vi "IPI_Cal_Step1.vi"(10 "Program":string(combo)="potteryTemplete", 11 "Image In":T2) -> (1 "Piex":string, 2 "result":string, 3 "Image Out":T2(plugin-control))   [LabVIEW 2015]
uses:
  <vilib>/vision/Image Controls.llb/IMAQ Image.ctl
  Global System.vi
  <vilib>/Utility/file.llb/Read Delimited Spreadsheet (string).vi
  <vilib>/vision/driver/NI_Vision_Acquisition_Software.lvlib
  <vilib>/Analysis/NI_AALPro.lvlib
panel:
  out "数字":i32[](array[numeric])
  out "all rows":string[][](array[string]) caption="所有行"
  out "Straight Edge (Find Straight Edge 1) 2":T1 {"Point2 (Real-World)"."Y" format="%.2f"; "Point2 (Real-World)"."X" format="%.2f"; "Point1 (Real-World)"."Y" format="%.2f"; "Point1 (Real-World)"."X" format="%.2f"; "Point2 (Pixels)"."Y" format="%.2f"; "Point2 (Pixels)"."X" format="%.2f"; "Point1 (Pixels)"."Y" format="%.2f"; "Point1 (Pixels)"."X" format="%.2f"}
  out "输出簇":cluster{"X":i32, "Y":i32}
  out "Dist piex":dbl
  out "y 焦点":dbl
  out "X 焦点":dbl
  out "b2":dbl
  out "k2":dbl
  out "元素":cluster{"X":dbl, "Y":dbl}
  out "数组":dbl[](array[numeric])
  out "大小":i32
  out "Contour Points (Contour Analysis 1)":cluster{"X":dbl, "Y":dbl}[](array[cluster])
  out "b1":dbl caption="截距"
  out "k1":dbl caption="斜率"
  in  "error in":errorcluster
  out "Straight Edge (Find Straight Edge 1)":T1 {"Point2 (Real-World)"."Y" format="%.2f"; "Point2 (Real-World)"."X" format="%.2f"; "Point1 (Real-World)"."Y" format="%.2f"; "Point1 (Real-World)"."X" format="%.2f"; "Point2 (Pixels)"."Y" format="%.2f"; "Point2 (Pixels)"."X" format="%.2f"; "Point1 (Pixels)"."Y" format="%.2f"; "Point1 (Pixels)"."X" format="%.2f"}
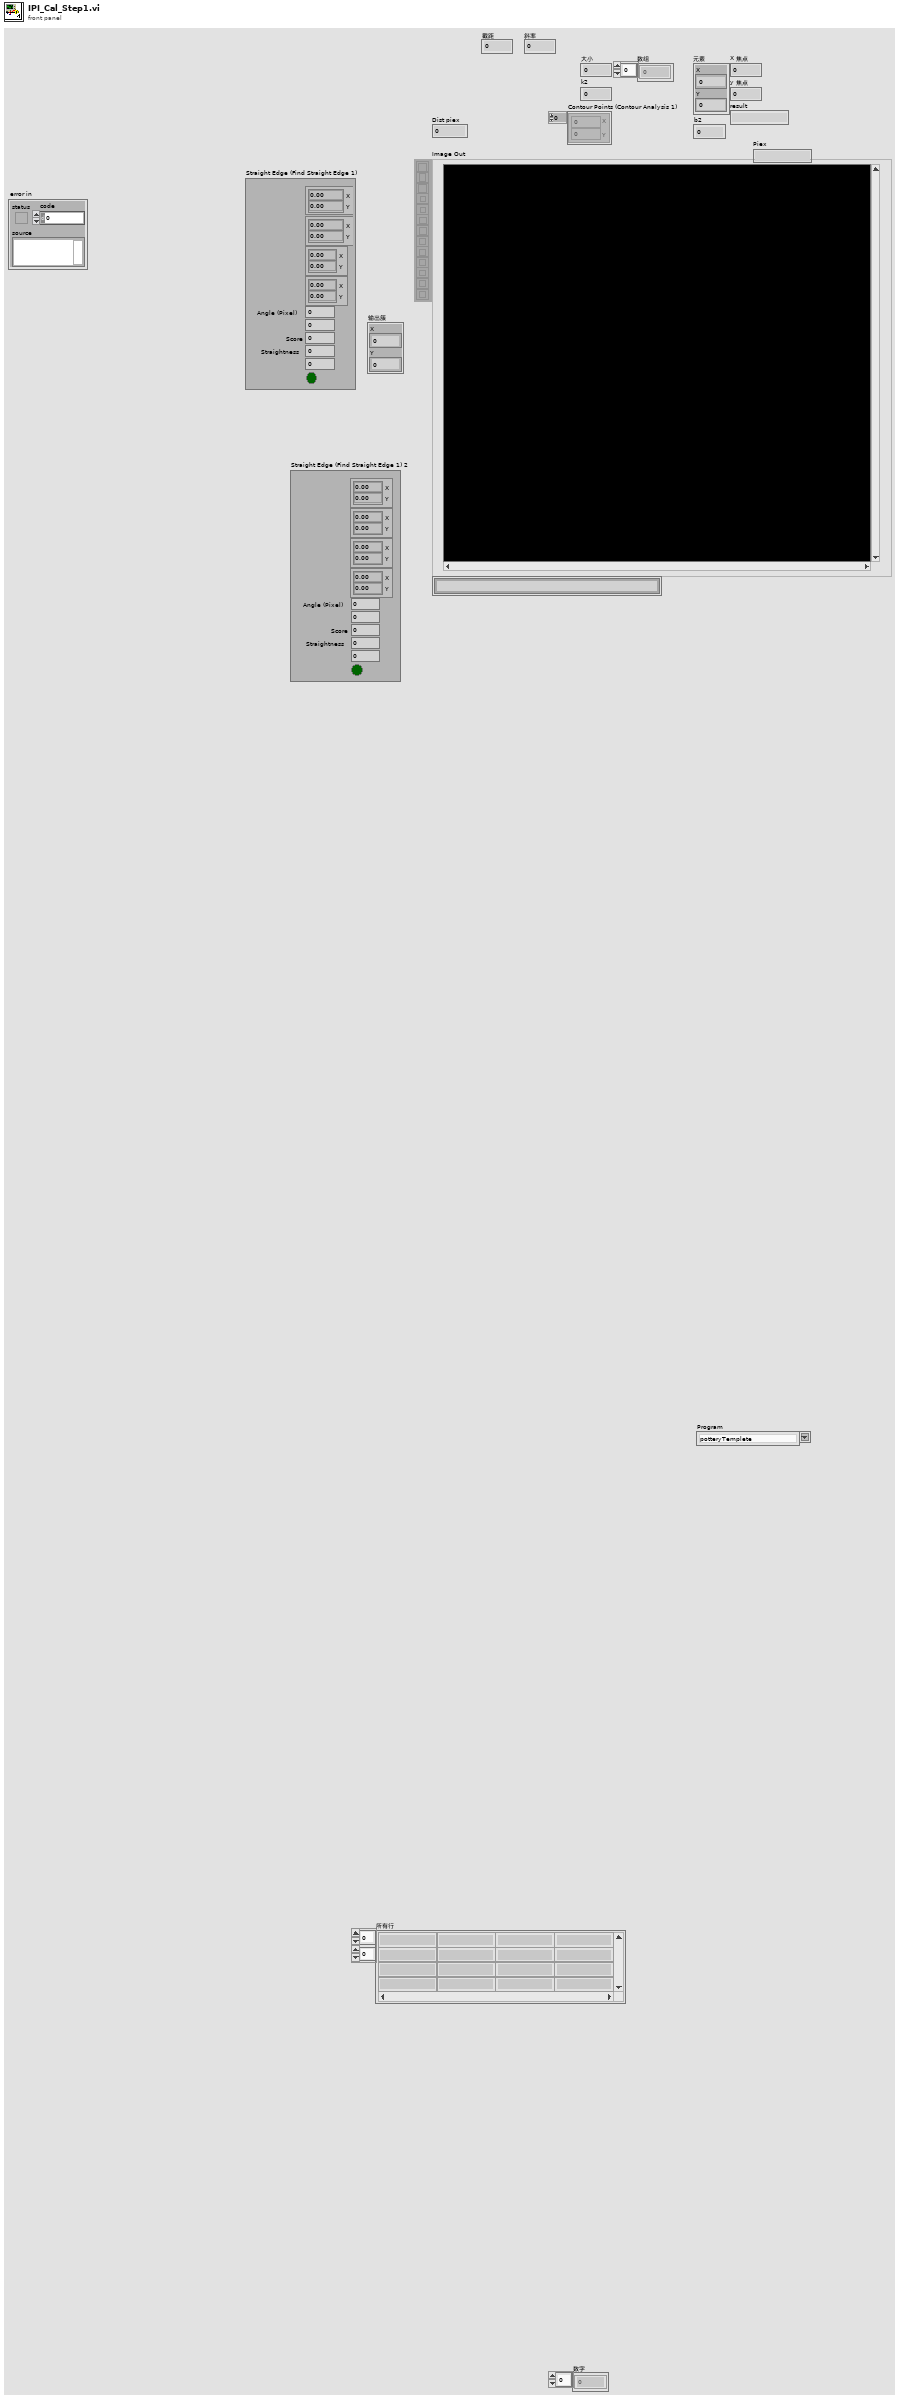
[diagram p1: front panel]
types:
  T1 = cluster{"Point1 (Pixels)":cluster{"X":sgl, "Y":sgl}, "Point2 (Pixels)":cluster{"X":sgl, "Y":sgl}, "Point1 (Real-World)":cluster{"X":sgl, "Y":sgl}, "Point2 (Real-World)":cluster{"X":sgl, "Y":sgl}, "Angle (Pixel)":dbl, "Angle (Real-World)":dbl, "Score":dbl, "Straightness":dbl, "Average SNR (db)":dbl, "Calibration Valid":bool}
  T2 = typedef "IMAQ Image.ctl" = refnum<image>
  T3 = cluster{"ID":enum32{"External", "Internal"}, "Type":u32, "Coordinates":i32[]}
  T4 = cluster{"Global Rectangle":i32[], "Contours":cluster{"ID":enum32{"External", "Internal"}, "Type":u32, "Coordinates":i32[]}[]}
  T5 = typedef "IMAQdx.ctl" = refnum<k21>
  T6 = cluster{"ID":enum32{"External", "Internal"}, "Type":u32, "Coordinates":i32[]}[]
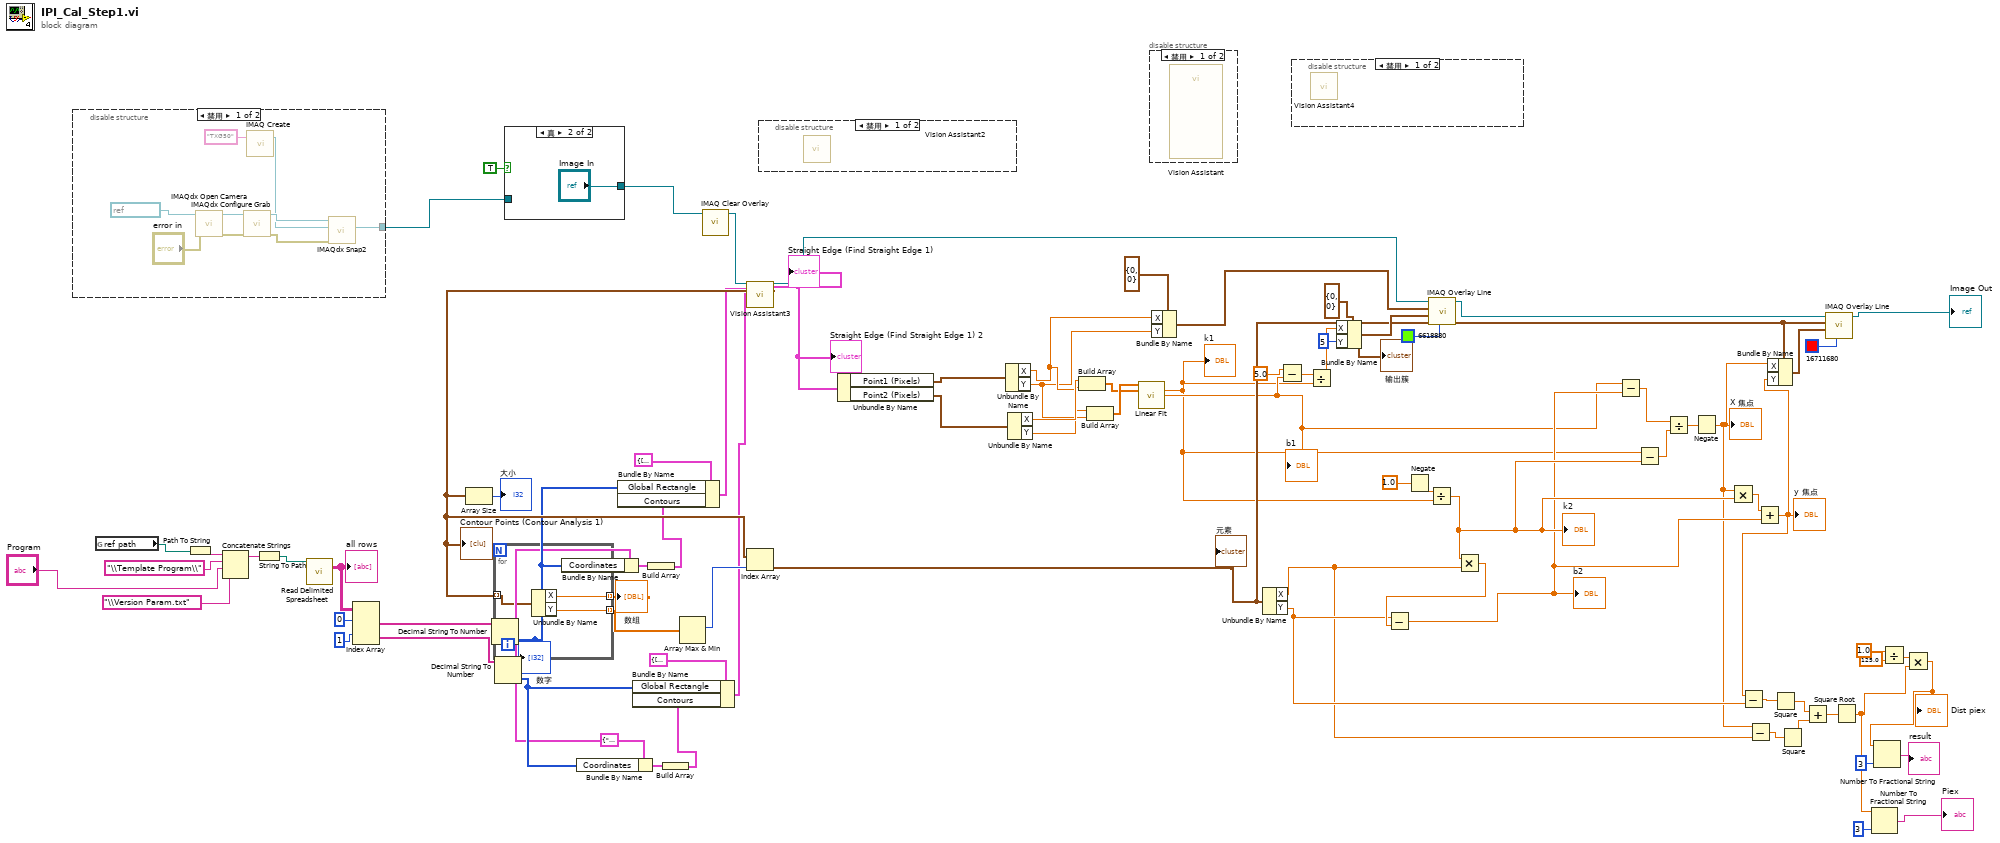
[diagram p0: block diagram]
diagram:
  w6 = T3 {"ID"=enum."External", "Type"=12, "Coordinates"=[983, 377, 1194, 1554, 1829]}
  n1 = disable-structure shown="禁用" {
    disable-tunnel: [w86 _] -> w4
    frame Disabled {
      n2 = call <vilib>:"IMAQdx Open Camera.vi"("error in"="error in", "Session In"=refnum<k21> "TXG50" ("Camera Name")) -> ("error out"=w94:errorcluster, "Session Out"=w93:T5)  [unwired: 1 in, 7 out]
      n3 = call <vilib>:"IMAQdx Configure Grab.vi"("error in"=w94, "Session In"=w93) -> ("error out"=w87:errorcluster, "Session Out"=w89:T5)  [unwired: 8 out]
      n4 = call "IMAQ Create"("Image Name"="TXG50") -> ("New Image"=w88:T2)  [unwired: 4 in, 1 out]
      n5 = call <vilib>:"IMAQdx Snap2.vi"("error in"=w87, "Image In"=w88, "Session In"=w89) -> ("Image Out"=w86:T2)  [unwired: 6 in, 2 out]
    }
    frame Enabled {
    }
  }
  n6 = global read "Global System.vi" "ref path"() -> (w23:path)
  n7 = Path To String(path=w23) -> (string=w25:string)
  n8 = Concatenate Strings(w25, "\\Template Program\\" ("字符串"), "Program", "\\Version Param.txt" ("字符串")) -> (w24:string)
  n9 = String To Path(string=w24) -> (path=w19:path)
  n10 = call-poly <vilib>:"Read Delimited Spreadsheet.vi"("file path (dialog if empty)"=w19) -> ("all rows"=w17:string[][])  [unwired: 9 in, 5 out]
  "all rows" <- w17
  n11 = Index Array(array=w17, index (row) #1=0 ("索引 (行)"), index (row) #2=1 ("禁用的索引 (列)")) -> (element #1=w16:string[], element #2=w11:string[])  [unwired: 2 in]
  n12 = Decimal String To Number(string=w16) -> (number=w13:i32[])  [unwired: 2 in, 1 out]
  "数字" <- w13
  n13 = Decimal String To Number(string=w11) -> (number=w8:i32[])  [unwired: 2 in, 1 out]
  n14 = case shown="真" TRUE {
    tunnel: [w95 "Image In"] -> w33
    tunnel: w4 -> [w95 _]
    frame False {
    }
    frame True {
    }
  }
  n15 = Bundle By Name(cluster=w6, "Coordinates"=w13) -> (w15:T3)
  n16 = Bundle By Name(cluster=w6, "Coordinates"=w8) -> (w10:T3)
  n17 = Build Array(w15) -> (w14:T6)
  n18 = Bundle By Name(cluster=T4 {"Global Rectangle"=[964, 373, 1213, 1558], "Contours"=[{"ID"=enum."External", "Type"=12, "Coordinates"=[983, 377, 1194, 1554, 1829]}]} ("ROI Descriptor (Find Straight Edge 1)"), "Global Rectangle"=w13, "Contours"=w14) -> (w5:T4)
  n19 = Build Array(w10) -> (w7:T6)
  n20 = Bundle By Name(cluster=T4 {"Global Rectangle"=[964, 373, 1213, 1558], "Contours"=[{"ID"=enum."External", "Type"=12, "Coordinates"=[983, 377, 1194, 1554, 1829]}]} ("ROI Descriptor (Find Straight Edge 1)"), "Global Rectangle"=w8, "Contours"=w7) -> (w1:T4)
  n21 = call "IMAQ Clear Overlay"("Image"=w33) -> ("Image Out"=w29:T2)  [unwired: 9 in, 1 out]
  n22 = call "Vision Assistant3"("Image In"=w29, "ROI Descriptor (Find Straight Edge 1)"=w5, "ROI Descriptor (Contour Analysis 1)"=w1) -> ("Image Out"=w28:T2, "Straight Edge (Find Straight Edge 1)"=w27:T1, "Contour Points (Contour Analysis 1)"=w26:cluster{"X":dbl, "Y":dbl}[])  [unwired: 19 in, 3 out]
  "Straight Edge (Find Straight Edge 1)" <- w27
  "Contour Points (Contour Analysis 1)" <- w26
  "Straight Edge (Find Straight Edge 1) 2" <- w27
  n23 = Array Size(array=w26) -> (size(s)=→"大小":i32)
  n24 = for {
    tunnel: w26 -> [w99] mode=indexing
    tunnel: [w98] -> w75 mode=indexing
    tunnel: [w97] -> w74 mode=indexing
    n25 = Unbundle By Name(w99) -> ("X"=w98:dbl, "Y"=w97:dbl)
  }
  "数组" <- w75
  n26 = Array Max & Min(array=w74) -> (max index (indices)=w73:i32)  [unwired: 3 out]
  n27 = Index Array(array=w26, index=w73) -> (element=w62:cluster{"X":dbl, "Y":dbl})
  "元素" <- w62
  n28 = disable-structure shown="禁用" {
    frame Disabled {
      n29 = call "Vision Assistant2"() -> ()  [unwired: 22 in, 6 out]
    }
    frame Enabled {
    }
  }
  n30 = Unbundle By Name(w27) -> ("Point1 (Pixels)"=w85:cluster{"X":sgl, "Y":sgl}, "Point2 (Pixels)"=w84:cluster{"X":sgl, "Y":sgl})
  n31 = Unbundle By Name(w85) -> ("X"=w42:sgl, "Y"=w40:sgl)
  n32 = Unbundle By Name(w84) -> ("X"=w43:sgl, "Y"=w41:sgl)
  n33 = Build Array(w43, w42) -> (w82:sgl[])
  n34 = Build Array(w41, w40) -> (w83:sgl[])
  n35 = call <vilib>:"Linear Fit.vi"("Y"=w83, "X"=w82) -> ("slope"=w36:dbl, "intercept"=w38:dbl)  [unwired: 9 in, 3 out]
  "k1" <- w36
  "b1" <- w38
  n36 = disable-structure shown="禁用" {
    frame Disabled {
      n37 = call "Vision Assistant"() -> ()  [unwired: 22 in, 6 out]
    }
    frame Enabled {
    }
  }
  n38 = Bundle By Name(cluster=cluster{"X":i32, "Y":i32} {"X"=0, "Y"=0} ("Start Point"), "X"=w42, "Y"=w40) -> (w78:cluster{"X":i32, "Y":i32})
  n39 = Unbundle By Name(w62) -> ("X"=w54:dbl, "Y"=w57:dbl)
  n40 = Subtract(x=5.0 ("y"), y=w38) -> (x-y=w37:dbl)
  n41 = disable-structure shown="禁用" {
    frame Disabled {
      n42 = call "Vision Assistant4"() -> ()  [unwired: 22 in, 6 out]
    }
    frame Enabled {
    }
  }
  n43 = Divide(x=w37, y=w36) -> (x/y=w35:dbl)
  n44 = Bundle By Name(cluster=cluster{"X":i32, "Y":i32} {"X"=0, "Y"=0} ("Start Point"), "X"=w35, "Y"=5) -> (w77:cluster{"X":i32, "Y":i32})
  "输出簇" <- w77
  n45 = Negate(x=1.0) -> (-x=w71:dbl)
  n46 = Divide(x=w71, y=w36) -> (x/y=w66:dbl)
  "k2" <- w66
  n47 = call "IMAQ Overlay Line"("Color"=u32 6618880, "End Point"=w77, "Start Point"=w78, "Image"=w28) -> ("Image Out"=w63:T2)  [unwired: 6 in, 1 out]
  n48 = Multiply(x=w66, y=w54) -> (x*y=w70:dbl)
  n49 = Subtract(x=w57, y=w70) -> (x-y=w64:dbl)
  "b2" <- w64
  n50 = Subtract(x=w38, y=w64) -> (x-y=w69:dbl)
  n51 = Subtract(x=w36, y=w66) -> (x-y=w68:dbl)
  n52 = Divide(x=w69, y=w68) -> (x/y=w67:dbl)
  n53 = Negate(x=w67) -> (-x=w55:dbl)
  "X 焦点" <- w55
  n54 = Multiply(x=w55, y=w66) -> (x*y=w65:dbl)
  n55 = Subtract(x=w55, y=w54) -> (x-y=w53:dbl)
  n56 = Add(x=w65, y=w64) -> (x+y=w58:dbl)
  "y 焦点" <- w58
  n57 = Subtract(x=w58, y=w57) -> (x-y=w56:dbl)
  n58 = Bundle By Name(cluster=w62, "X"=w55, "Y"=w58) -> (w61:cluster{"X":dbl, "Y":dbl})
  n59 = Square(x=w56) -> (x^2=w52:dbl)
  n60 = Square(x=w53) -> (x^2=w51:dbl)
  n61 = Add(x=w52, y=w51) -> (x+y=w50:dbl)
  n62 = call "IMAQ Overlay Line"("Color"=u32 16711680, "End Point"=w61, "Start Point"=w62, "Image"=w63) -> ("Image Out"=→"Image Out":T2)  [unwired: 6 in, 1 out]
  n63 = Square Root(x=w50) -> (sqrt(x)=w31:dbl)
  n64 = Number To Fractional String(number=w31, precision (6)=i16 3 ("精度(6)")) -> (F-format string=→"Piex":string)  [unwired: 2 in]
  n65 = Divide(x=1.0, y=125.0) -> (x/y=w45:dbl)
  n66 = Multiply(x=w45, y=w31) -> (x*y=w44:dbl)
  "Dist piex" <- w44
  n67 = Number To Fractional String(number=w44, precision (6)=i16 3 ("精度(6)")) -> (F-format string=→"result":string)  [unwired: 2 in]
